vi "Get Protocol Type.vi"(8 "error in (no error)":errorcluster, 11 "TCP in":refnum<class "TCP.lvclass">) -> (0 "error out":errorcluster, 2 "protocol type":T1=enum."AK RS-XXX", 3 "TCP out":refnum<class "TCP.lvclass">)   [LabVIEW 2018, in "Protocols.lvlib" / "TCP.lvclass"]
doc: "Returns TCP|IP protocol type Enum.\n\nInput:\nTCP in: represents an instance of the TCP protocol class.\n\nOutput: \nTCP out: represents an instance of the TCP protocol class provided as input.\nProtocol Type: represents the type of the protocol in Enum format."
uses:
  TCP.lvclass
  Protocol Parent/Types/Protocol Type.ctl
  Protocol Parent/Protocol Parent.lvclass
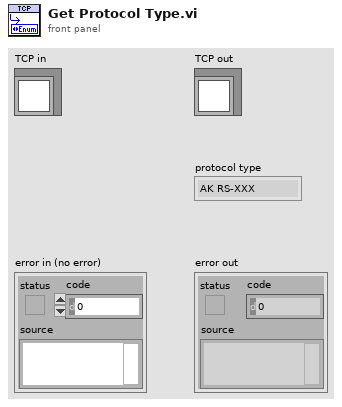
[diagram p1: front panel]
types:
  T1 = typedef "Protocols.lvlib/Protocol Parent.lvclass/Protocol Type.ctl" = enum16{"RS-XXX", "AK RS-XXX", "VISA", "TCPIP", "AK TCPIP", "UDP", "GPIB ConvBox"}
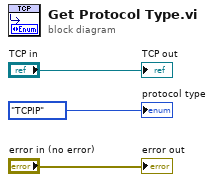
[diagram p0: block diagram]
diagram:
  "error out" <- "error in (no error)"
  "TCP out" <- "TCP in"
  "protocol type" <- Protocol_Type."TCPIP" ("Protocol out")
